vi "RD Digital In Status.vi"(8 "error in (no error)":errorcluster caption="错误输入（无错误）", 11 "handle":u64) -> (0 "error out":errorcluster caption="错误输出", 1 "function return":i32, 2 "sts out":u8, 3 "handle out":u64)   [LabVIEW 2018, in "InstrumentsPlayground.lvlib"]
doc: "CLIFFAPI int CliffDigitalInStatus(FT_HANDLE handle,CLIFFState* sts);\nconst CLIFFState CLIFFStateReady = 0;\nconst CLIFFState CLIFFStateConfig = 4;\nconst CLIFFState CLIFFStatePrefill = 5;\nconst CLIFFState CLIFFStateArmed = 1;\nconst CLIFFState CLIFFStateWait = 7;\nconst CLIFFState CLIFFStateTriggered = 3;\nconst CLIFFState CLIFFStateRunning = 3;\nconst CLIFFState CLIFFStateDone = 2;s"
uses:
  InstrumentsPlayground.lvlib
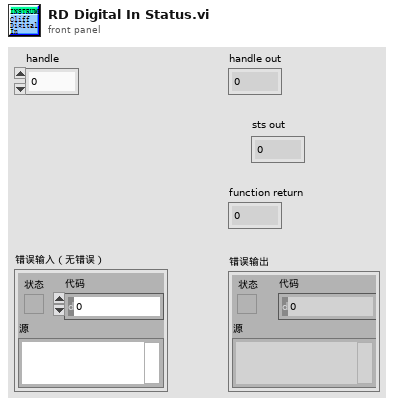
[diagram p1: front panel]
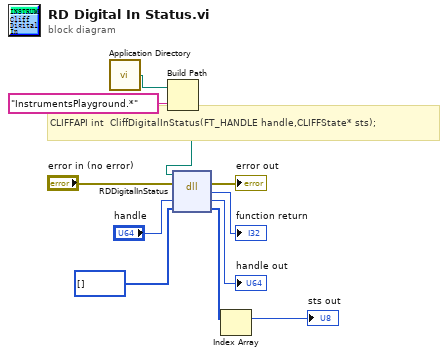
[diagram p0: block diagram]
diagram:
  # "CLIFFAPI int  CliffDigitalInStatus(FT_HANDLE handle,CLIFFState* sts);"
  n1 = call <vilib>:"Application Directory.vi"() -> ("Application Directory"=w3:path)
  n2 = Build Path(base path=w3, name or relative path="InstrumentsPlayground.*" ("名称或相对路径")) -> (appended path=w2:path)
  n3 = dll-call lib="E:/work/YZCourse_Xtext/Cliff/API/LabVIEW lib/InstrumentsPlayground.*" fn="RDDigitalInStatus"(path in=w2, error in="error in (no error)", "handle"="handle", "sts"=i32[] []) -> (error out=→"error out":errorcluster, "返回类型"=→"function return":i32, "handle"=→"handle out":u32, "sts"=w7:u8[])  [unwired: 1 in, 1 out]
  n4 = Index Array(array=w7) -> (element=→"sts out":u8)  [unwired: 1 in]
